vi "Read_File+_[U16].ph.vi"(6 "2D number of columns/1D count":i32, 7 "2D number of rows":i32, 8 "error in (no error)":errorcluster, 9 "pos offset (bytes:0)":i32, 10 "pos mode (rel. to current:2)":enum16{"start", "end", "current"}(ring)=enum."current", 11 "refnum":refnum<file>) -> (0 "error out":errorcluster, 1 "mark after read (bytes)":i32, 2 "1D data":u16[](array[numeric]), 3 "2D data":u16[][](array[numeric]), 4 "EOF?":bool, 5 "dup refnum":refnum<file>)   [LabVIEW 2010]
doc: "Reads a 2D or 1D array of signed word integers (I16) from a byte stream file at the specified location; the default location is at the current mark. The VI does incoming and internal error checking and does not read if an incoming error occurs.\n\nrefnum is the reference number of the open file.\n\npos mode specifies where the write begins relative to pos offset:\n\n 0: at the beginning of the file plus pos offset.\n\n 1: at the end of the file plus pos offset. \n\n 2: at the current file mark plus pos offset. This is the default value.\n\npos offset specifies in bytes how far from the location specified by pos mode that the operation begins. The default value is 0. Byte units rather than integer (2 byte) units for flexibility, for example, so that a file can contain a text header written with Write File+ (string) followed by arrays of number written with Write File+ [I16].\n\n2D number of rows is the number of rows to create if the data is to be returned in the 2D array output. If the value is 0 (default), the data is returned in the 1D array.\n\n2D number of columns/1D count is the number of columns to create if the data is to be returned in the 2D array output, provided that 2D number of rows is >0; otherwise, this is the number of signed word integers to read and return in the 1D array output.\n\nerror in is a cluster of three elements (error?, code, and source) that describe the upstream error state, that is, the existance of any error preceeding the execution of the VI. The VI executes normally only if no incoming error exists; otherwise it merely passes the error in value to error out. error? is TRUE if an error occurred; the default value is FALSE. code is the error code; the default value is 0. source is in most cases the name of the VI or function that produced the error; the default value is an empty string.\n\ndup refnum is a flow-though parameter with the same value as refnum.\n\n2D array contains the signed word integers read from the file if 2D number of rows is greater than 0; otherwise, this output is empty.\n\n1D array contains the signed word integers read from the file if 2D number of rows equal 0; otherwise, this output is empty.\n\nmark after read is the location of the file mark after the read; it points to the byte in the file following the last byte read.\n\nEOF? is TRUE if you attempt to read past the end of file.\n\nerror out is a cluster of three elements (error?, code, and source) that describe the error state following the execution of the VI. If an incoming error does not exist, the VI executes normally and error out describes the VI's error state; if an incoming error exists, error out equals error in."
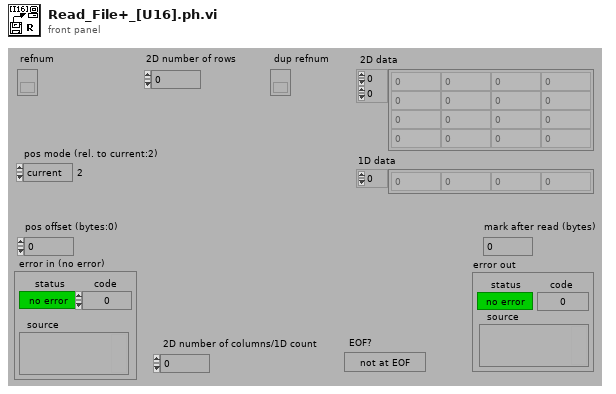
[diagram p1: front panel]
types:
  T1 = cluster{"2D number of rows":i32, "2D number of columns/1D count":i32}
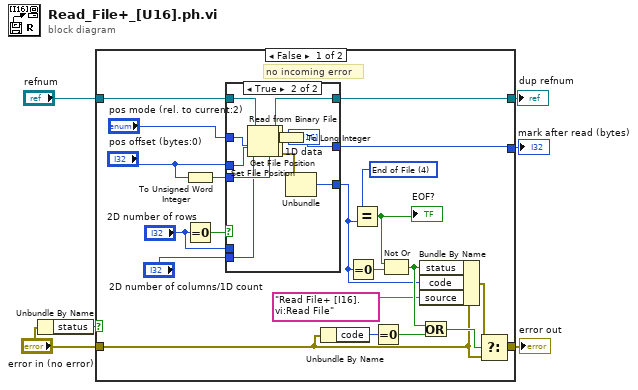
[diagram p0: block diagram]
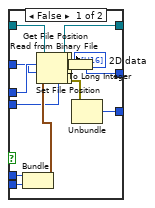
[diagram p2: hidden frame]
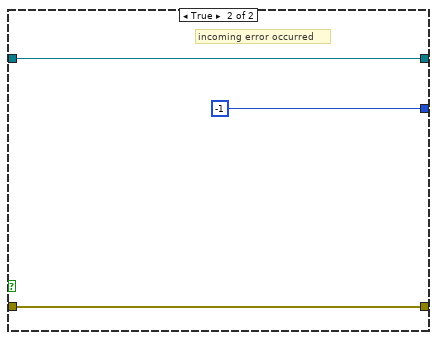
[diagram p3: hidden frame]
diagram:
  n1 = Unbundle By Name("error in (no error)") -> ("status"=w6:bool)
  n2 = case shown="False" w6 {
    tunnel: [w8 w61] -> w5
    tunnel: [w20 -1] -> w4
    tunnel: [w25 w60] -> w3
    tunnel: "refnum" -> [w24 w60]
    tunnel: "error in (no error)" -> [w12 w61]
    frame False {
      w7 = 4 items=["No Error", "Manager Argument Error", "Memory Full", "Out of Zone", "End of File", "File Already Open", "Generic File IO Error", "File Not Found", "File Permission Error", "Disk Full", "Duplicate Path", "Too Many Files Open", "Not Enabled", "Resource File Not Found", "Cannot Add Resource", "Resource Not Found", "Image Not Found", "Image Memory Error", "Pen Does Not Exist", "Config Bad Type", "Config Token Not Found", "Config Parse Error", "Config Memory Error", "Bad External Code Format", "Bad External Code Offset", "External Code Not Present", "Null Window", "Destroy Window Mixup", "Null Menu", "Print Aborted", "Bad Print Record", "Print Driver Error", "Windows Error During Print", "Memory Error During Print", "Print Dialog Error", "Generic Print Error", "Invalid Device Refnum", "Device Not Found", "Device Parameter Error", "Device Unit Error", "Can't Open Device", "Device Call Aborted", "Generic Error", "Cancelled By User", "Object ID Too Low", "Object ID Too High", "Object Not In Heap", "Unknown Heap", "Bad DefProc ID", "DefProc Not In Table", "Message Out Of Range", "Null Method", "Unknown Message", "Manager Call Not Supported"]
      # "no incoming error"
      n3 = To Unsigned Word Integer(number="pos offset (bytes:0)") -> (unsigned 16bit integer=w27:u16)
      n4 = Equal To 0?(x="2D number of rows") -> (x = 0?=w26:bool)
      n5 = case shown="True" w26 {
        tunnel: [w35 w52] -> w10
        tunnel: [w39 w59] -> w20
        tunnel: w27 -> [w43 w58]
        tunnel: "2D number of columns/1D count" -> [w42 w53]
        tunnel: "2D number of rows" -> [w41 _]
        tunnel: [w38 w55] -> w25
        tunnel: w24 -> [w37 w56]
        tunnel: "pos mode (rel. to current:2)" -> [w33 w50]
        tunnel: "pos offset (bytes:0)" -> [w36 w54]
        frame False {
          n6 = Bundle("2D number of rows"=w41, "2D number of columns/1D count"=w42) -> (w44:T1)  [unwired: 1 out]
          n7 = Set File Position(offset (in bytes) (0)=w36, refnum=w37, from (0:start)=w33) -> (refnum out=w32:refnum<file>, error out=w31:errorcluster)  [unwired: 1 in]
          n8 = Read from Binary File(5:w43, 8:w31, 10:w44, 11:w32) -> (0:w29:errorcluster, 2:→"2D data":u16[][], 3:w30:refnum<file>)  [unwired: 3 out]
          n9 = Get File Position(4:w29, 7:w30) -> (0:w34:errorcluster, 2:w28:i64, 3:w38:refnum<file>)
          n10 = To Long Integer(number=w28) -> (32bit integer=w39:i32)
          n11 = Unbundle(w34) -> ("code"=w35:i32)  [unwired: 2 out]
        }
        frame True {
          n12 = Set File Position(offset (in bytes) (0)=w54, refnum=w56, from (0:start)=w50) -> (refnum out=w49:refnum<file>, error out=w48:errorcluster)  [unwired: 1 in]
          n13 = Read from Binary File(5:w58, 8:w48, 10:w53, 11:w49) -> (0:w46:errorcluster, 2:→"1D data":u16[], 3:w47:refnum<file>)  [unwired: 3 out]
          n14 = Get File Position(4:w46, 7:w47) -> (0:w51:errorcluster, 2:w45:i64, 3:w55:refnum<file>)
          n15 = To Long Integer(number=w45) -> (32bit integer=w59:i32)
          n16 = Unbundle(w51) -> ("code"=w52:i32)  [unwired: 2 out]
        }
      }
      n17 = Unbundle By Name(w12) -> ("code"=w16:i32)
      n18 = Equal To 0?(x=w10) -> (x = 0?=w18:bool)
      n19 = Equal?(x=w7, y=w10) -> (x = y?=w11:bool)
      "EOF?" <- w11
      n20 = Equal To 0?(x=w16) -> (x = 0?=w14:bool)
      n21 = Not Or(1:w18, 2:w11) -> (0:w15:bool)
      n22 = Bundle By Name(cluster=w12, "status"=w15, "code"=w10, "source"="Read File+ [I16].vi:Read File") -> (w17:errorcluster)
      n23 = Or(x=w15, y=w14) -> (x .or. y?=w13:bool)
      n24 = Select(t=w17, s=w13, f=w12) -> (s? t:f=w8:errorcluster)
    }
    frame True {
      # "incoming error occurred"
    }
  }
  "error out" <- w5
  "mark after read (bytes)" <- w4
  "dup refnum" <- w3
